vi "Populate Tree.vi"(7 "Results":map{path, string}(c390), 8 "error in (no error)":errorcluster, 9 "VIs":set{path}(c389), 10 "Project Path":path, 11 "TreeControl in":refnum<vi>) -> (0 "error out":errorcluster)   [LabVIEW 2020, in "Coverage Report.lvclass"]
uses:
  Coverage Report.lvclass
  Tree Helpers/File Tree/File Tree.lvclass
  Tree Helpers/File Tree/File Tree.lvclass/File Tree.ctl
  Coverage Report.lvclass/Coverage Report.ctl
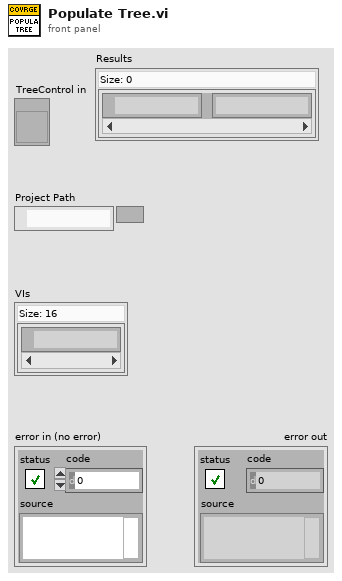
[diagram p1: front panel]
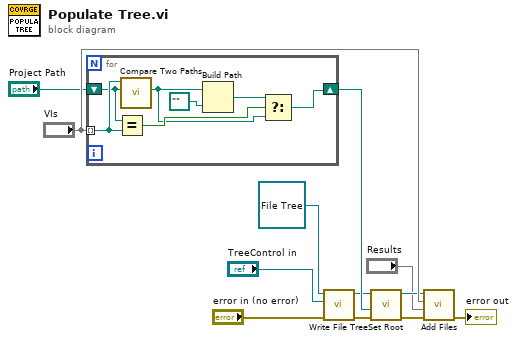
[diagram p0: block diagram]
diagram:
  n1 = for {
    tunnel: "VIs" -> [w19] mode=indexing
    shift-right: [w16] -> w12
    shift-left: "Project Path" -> [w18]
    n2 = Equal?(x=w18, y=w19) -> (x = y?=w17:bool)
    n3 = call <vilib>:"Compare Two Paths.vi"("Path 2"=w18, "Path 1"=w19) -> ("Common Path"=w14:path)  [unwired: 6 in, 3 out]
    n4 = Build Path(base path=w14, name or relative path=path "..") -> (appended path=w15:path)
    n5 = Select(t=w15, s=w17, f=w14) -> (s? t:f=w16:path)
  }
  n6 = call "Write File Tree.vi"("error in (no error)"="error in (no error)", "File Tree Reference"="TreeControl in", "File Tree In"=refnum<class "File Tree.lvclass"> refnum ("Support Utilities.lvlib:Tag Tree.lvclass")) -> ("error out"=w7:errorcluster, "File Tree Out"=w5:refnum<class "File Tree.lvclass">)  [unwired: 7 in]
  n7 = call "Set Root.vi"("error in (no error)"=w7, "Root Path"=w12, "File Tree In"=w5) -> ("error out"=w8:errorcluster, "File Tree Out"=w6:refnum<class "File Tree.lvclass">)  [unwired: 7 in]
  n8 = call "Add Files.vi"("error in (no error)"=w8, "Results"="Results", "Files"="VIs", "File Tree In"=w6) -> ("error out"=→"error out":errorcluster)  [unwired: 6 in, 1 out]
